vi "Harvest Arm.vi"(9 "Arm Down":bool, 11 "Arm Up":bool) -> ()   [LabVIEW 2015]
panel:
  in  "Harvester Arm Setpoint Up":dbl=0.53 format="%.2f"
  in  "Harvester Arm Setpoint Down":dbl=0.22 format="%.2f"
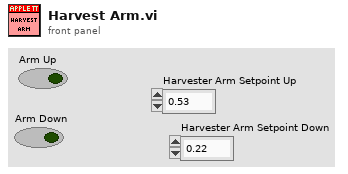
[diagram p1: front panel]
types:
  T1 = typedef "WPI_MotorControlDeviceRef.ctl" = cluster{"DeviceStatus":errorcluster, "Type":T2, "PWM":cluster{"PWM Channel":T3, "DeadBand":T4}, "CAN":cluster{"Device Number":u8, "Control Mode":T5, "Semaphore":T6, "Max Vout":dbl, "TalonSRX Control Mode":T7}, "Invert":bool}
  T2 = typedef "WPI_MotorControlType.ctl" = enum16{"PWM", "CAN", "CANTalonSRX"}
  T3 = typedef "FPGA_DIOPWMChannel.ctl" = enum8{"PWM 0", "PWM 1", "PWM 2", "PWM 3", "PWM 4", "PWM 5", "PWM 6", "PWM 7", "PWM 8", "PWM 9", "PWM MXP 0", "PWM MXP 1", "PWM MXP 2", "PWM MXP 3", "PWM MXP 4", "PWM MXP 5", "PWM MXP 6", "PWM MXP 7", "PWM MXP 8", "PWM MXP 9", "Invalid"}
  T4 = typedef "WPI_PWMDeadband.ctl" = cluster{"Name":string, "maxPositivePwm":i32, "minPositivePwm":i32, "centerPwm":i32, "maxNegativePwm":i32, "minNegativePwm":i32, "angularRange":u16}
  T5 = typedef "WPI_CANJaguar_ControlMode.ctl" = enum8{"Percent VBus", "Current", "Speed", "Position", "Voltage"}
  T6 = typedef "Semaphore RefNum" = refnum<k1>
  T7 = typedef "WPI_CANTalonSRX_APIControlMode.ctl" = enum8{"Percent VBus", "Speed", "Position", "Slave", "Unchanged / Invalid", "Voltage Compensation", "Current", "Motion Profile"}
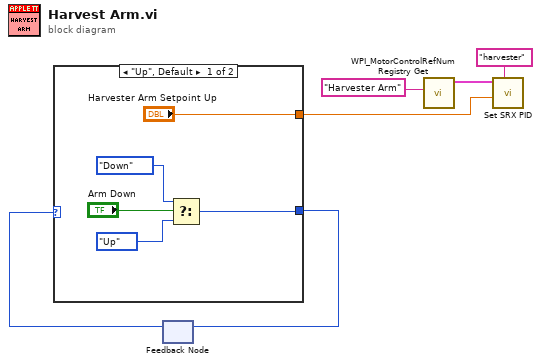
[diagram p0: block diagram]
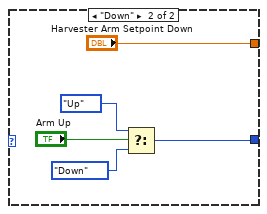
[diagram p2: hidden frame]
diagram:
  n1 = feedback #1() -> (w5:enum16{"Up", "Down"})  [unwired: 1 in]
  n2 = case shown="\"Up\", Default" w5 {
    tunnel: [w8 w14] -> w6
    tunnel: ["Harvester Arm Setpoint Up" "Harvester Arm Setpoint Down"] -> w4
    frame "Up", Default {
      n3 = Select(t=enum16{"Up", "Down"}."Down", s="Arm Down", f=enum16{"Up", "Down"}."Up") -> (s? t:f=w8:enum16{"Up", "Down"})
    }
    frame "Down" {
      n4 = Select(t=enum16{"Up", "Down"}."Up", s="Arm Up", f=enum16{"Up", "Down"}."Down") -> (s? t:f=w14:enum16{"Up", "Down"})
    }
  }
  n5 = feedback-in #1(w6) -> ()
  n6 = call <vilib>:"WPI_MotorControlRefNum Registry Get.vi"("refnum name"="Harvester Arm") -> ("MotorControlDevRef"=w2:T1)  [unwired: 9 in, 1 out]
  n7 = call "Set SRX PID.vi"("subsystem"="harvester", "Setpoint"=w4, "CAN Talon SRX Ref"=w2) -> ()  [unwired: 8 in, 1 out]
